vi "R=Table.vi"(6 "picture":refnum<vi>, 8 "Offset":T4, 9 "Matrix":T3 format="%.3f", 11 "Command":string="Save") -> (0 "error out":errorcluster, 2 "Joints":dbl[](array[numeric]), 3 "Pose Out":T3 format="%.3f")   [LabVIEW 2013]
uses:
  <vilib>/Analysis/Matrix/Datatypes/RealMatrix.ctl
  ROS/Code/SubVIs/BaxterSide.ctl
  Teach Locations.ctl
  ROS/Code/Console/Servers/ServerSubs/(nist) Arm Globals.vi
  Arm Globals.vi
  <vilib>/Analysis/baseanly.llb/Real Inverse Matrix.vi
  <vilib>/Analysis/Matrix/Numeric/Conversions/Array To Matrix - RA.vi
  <vilib>/Analysis/Matrix/Numeric/Multiply/Multiply - RM,RM.vi
  Move/Move XYA.vi
  <vilib>/Utility/config.llb/Write Key (String).vi
  <vilib>/Utility/config.llb/Read Key (String).vi
  <vilib>/Analysis/NI_AALBase.lvlib
  <vilib>/Analysis/Matrix/NI_Matrix.lvlib
  <vilib>/Utility/config.llb/NI_LVConfig.lvlib
panel:
  in  "Tab Control":T1(tab)=enum."Calibration Table"
  out "picture 2":picture
  out "Progress":T2
  out "IK Found":bool=TRUE
  in  "Table":T5={"Far Left"={"Absolute"=[250.0, 545.0, 0.0, 0.0], "Robot"=[672.1715994990807, 48.007748317552725, 100.0, 20.0]}, "Far Right"={"Absolute"=[250.0, 25.0, 0.0, 0.0], "Robot"=[665.1874122546096, -469.0278466112149, 100.0, 20.0]}, "Near Left"={"Absolute"=[25.0, 545.0, 0.0, 0.0], "Robot"=[441.4908301445158, 48.901036437406674, 100.0, 20.0]}, "Near Right"={"Absolute"=[25.0, 25.0, 0.0, 0.0], "Robot"=[437.9607504937842, -467.7872050538727, 100.0, 20.0]}}
  in  "Reference":dbl[](array[numeric])=[44.89013666745554, -43.242187450588595, -0.1098632811244629, 63.3471678963653, 0.1318359373493555, 69.71923820158416, -0.021972656224892577]
  # "Basic Commands are:\n   Convert   - convert offset to joints\n   Current   - current joint and offset\n   Register  - determine position\n   Save      - save calibration data\n   Load      - load calibration data\n   Reference - give reference joint position"
  # "Position gripper over center before starting"
  # "Insert the Absolute Positions here before \nrunning registration\n\nRun \"Save\" to load this table.\nMust manual set current values to default\nand save the vi."
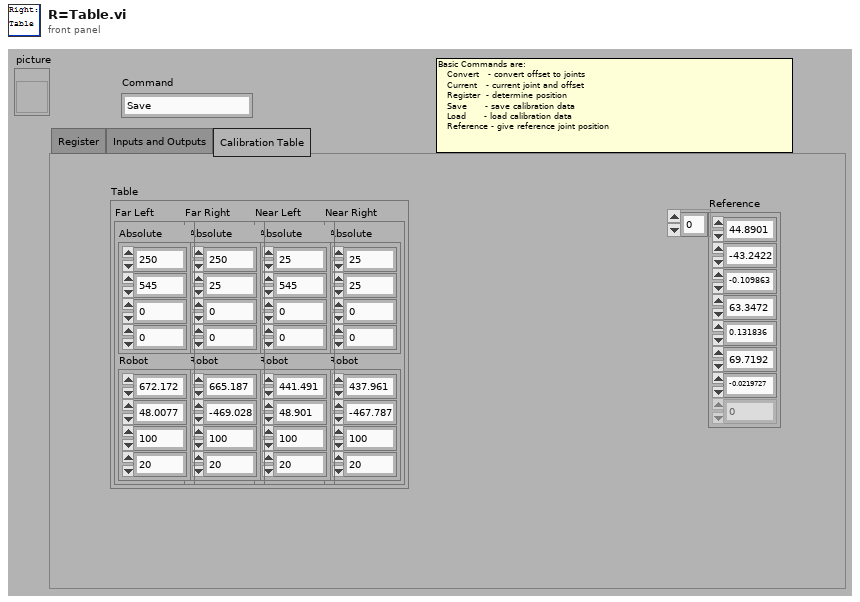
[diagram p1: front panel]
types:
  T1 = enum32{"Register", "Inputs and Outputs", "Calibration Table"}
  T2 = cluster{"1":bool, "1 2":bool, "1 3":bool, "1 4":bool}
  T3 = typedef "NI_Matrix.lvlib/RealMatrix.ctl" = dbl[][]
  T4 = cluster{"X":dbl, "Y":dbl, "Z":dbl, "Roll":dbl, "Pitch":dbl, "Yaw":dbl}
  T5 = cluster{"Far Left":cluster{"Absolute":dbl[], "Robot":dbl[]}, "Far Right":cluster{"Absolute":dbl[], "Robot":dbl[]}, "Near Left":cluster{"Absolute":dbl[], "Robot":dbl[]}, "Near Right":cluster{"Absolute":dbl[], "Robot":dbl[]}}
  T6 = typedef "BaxterSide.ctl" = enum16{"left", "right"}
  T7 = typedef "Teach Locations.ctl" = enum16{"Far_Right", "Near_Right", "Far_Left", "Near_Left", "Bottom", "Top", "Right", "Left"}
  T8 = typedef "NI_LVConfig.lvlib/Config Data RefNum.ctl" = refnum<k1>
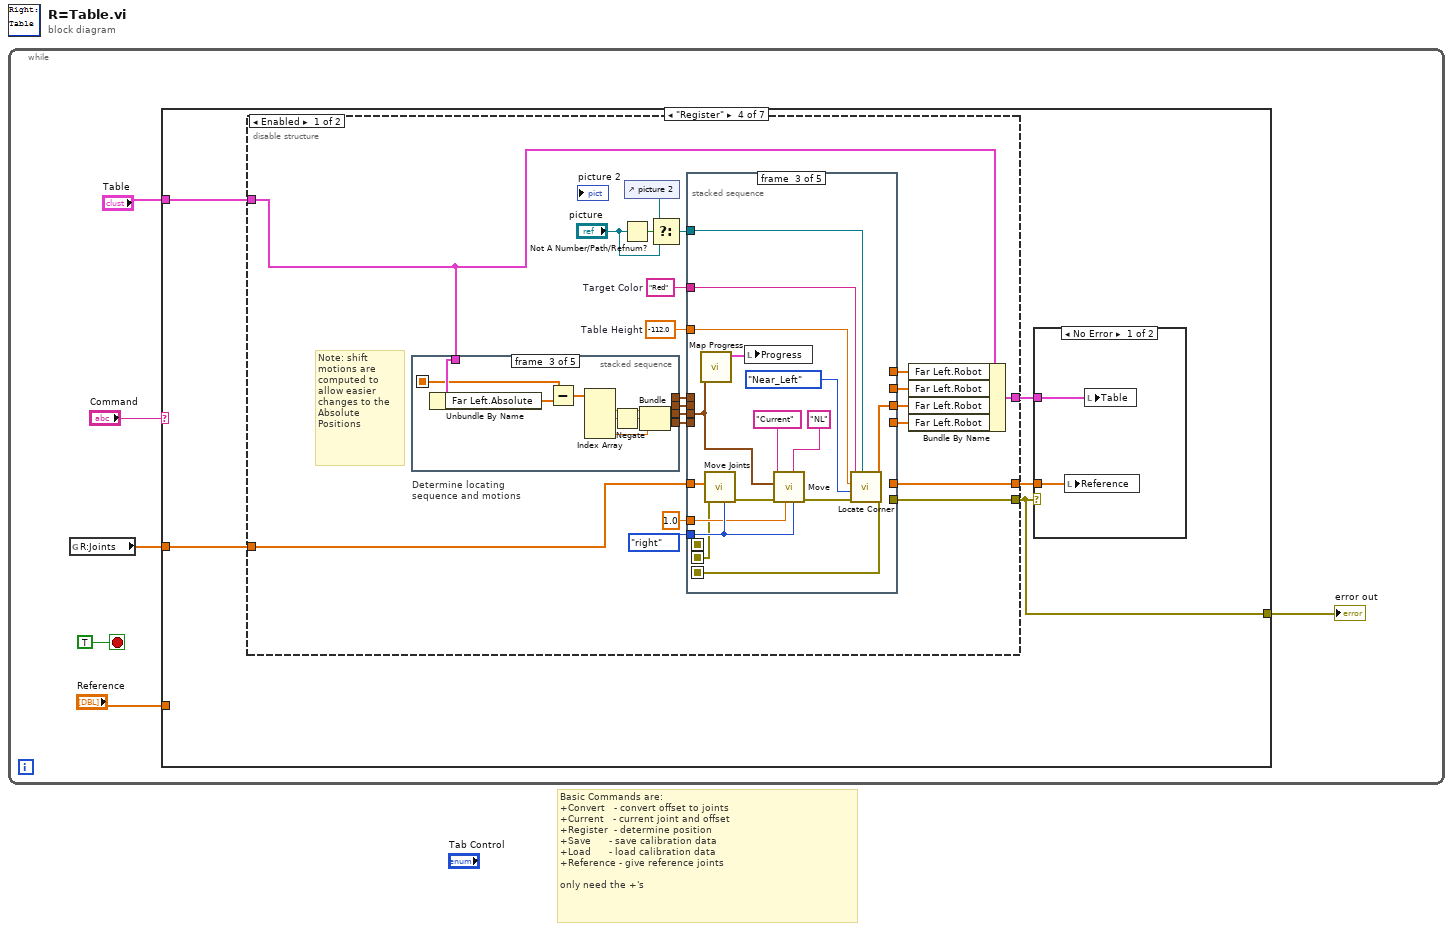
[diagram p0: block diagram]
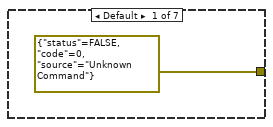
[diagram p2: hidden frame]
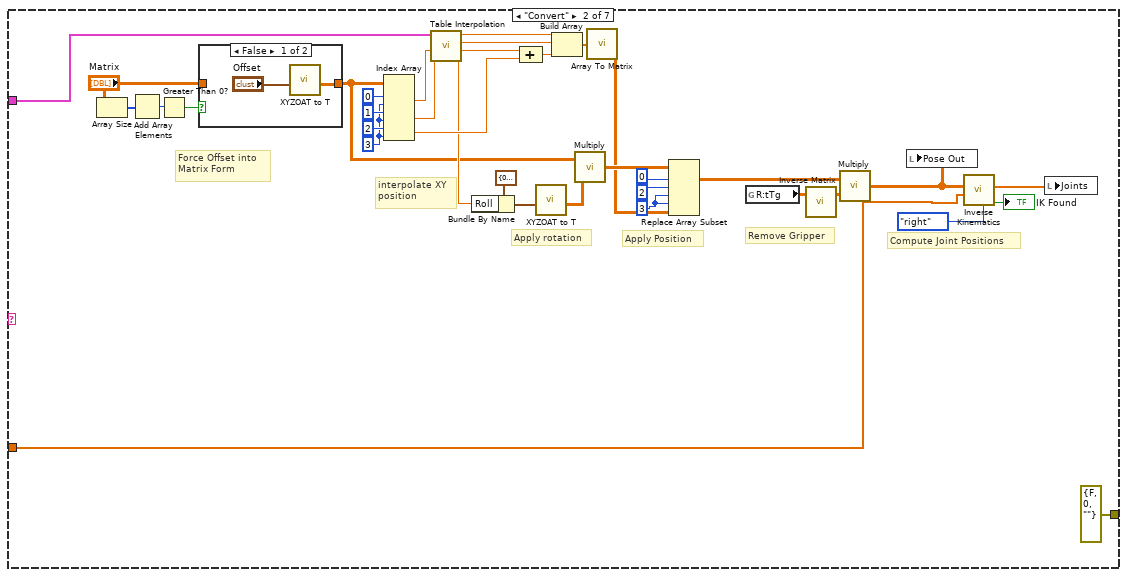
[diagram p3: hidden frame]
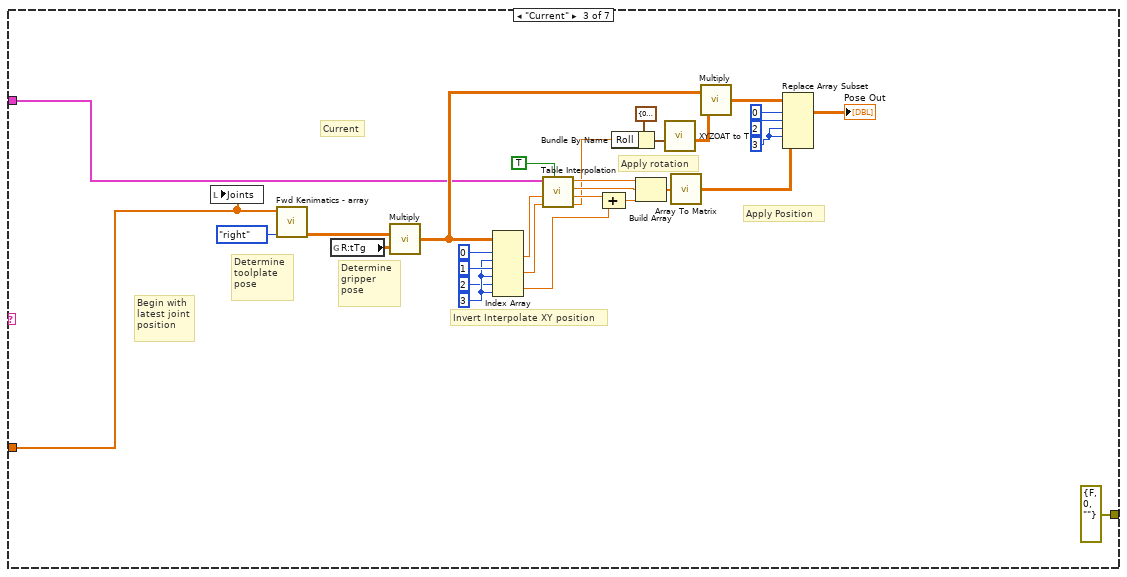
[diagram p5: hidden frame]
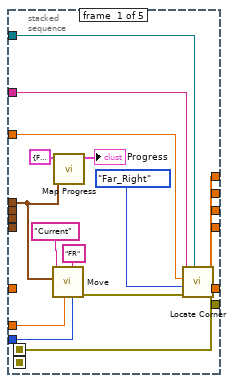
[diagram p6: hidden frame]
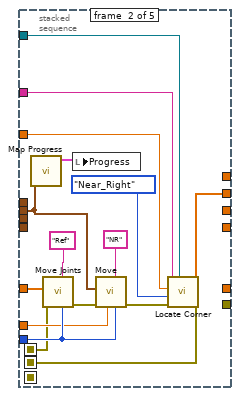
[diagram p7: hidden frame]
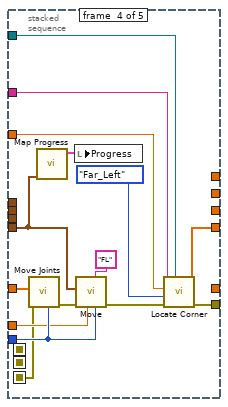
[diagram p8: hidden frame]
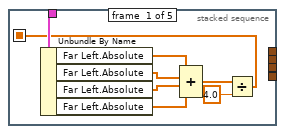
[diagram p10: hidden frame]
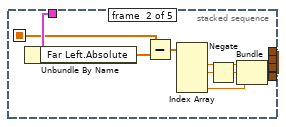
[diagram p11: hidden frame]
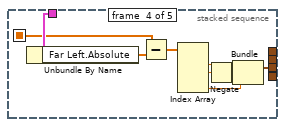
[diagram p12: hidden frame]
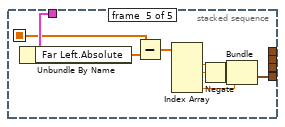
[diagram p13: hidden frame]
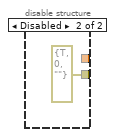
[diagram p14: hidden frame]
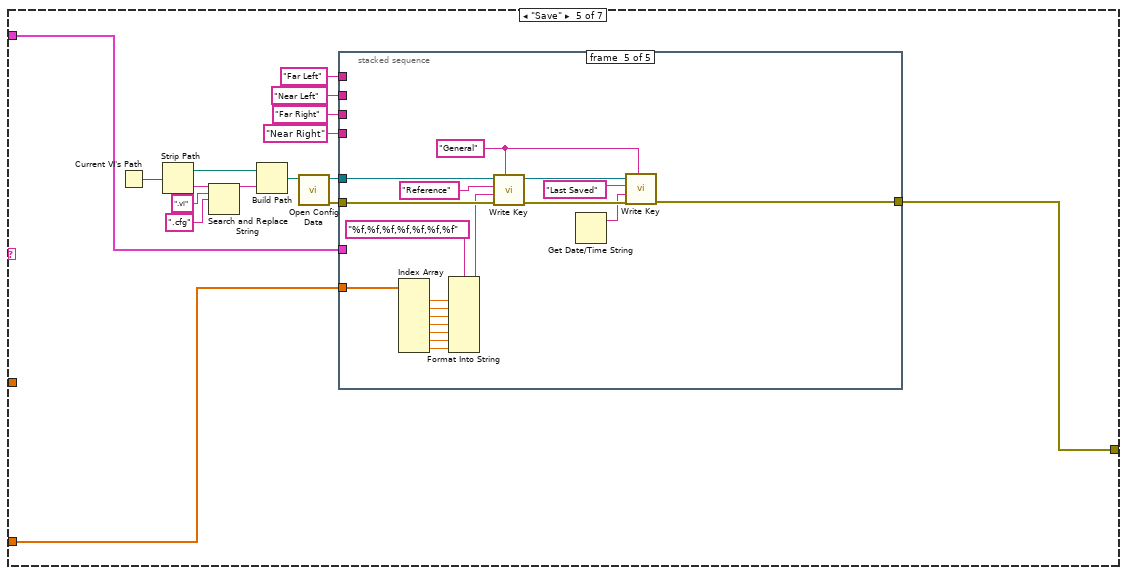
[diagram p16: hidden frame]
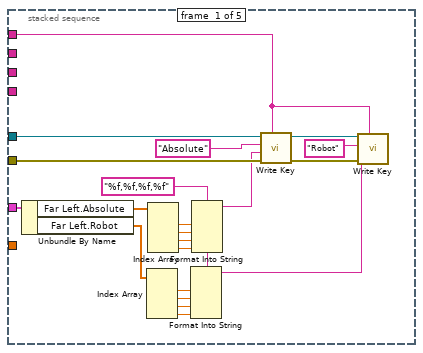
[diagram p17: hidden frame]
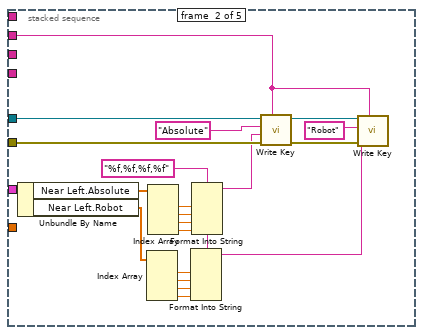
[diagram p18: hidden frame]
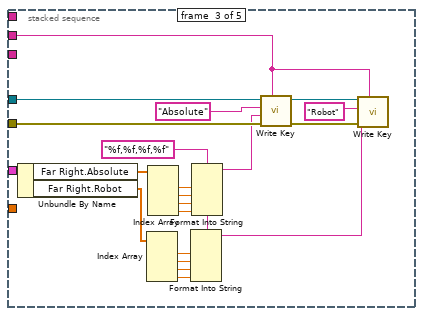
[diagram p19: hidden frame]
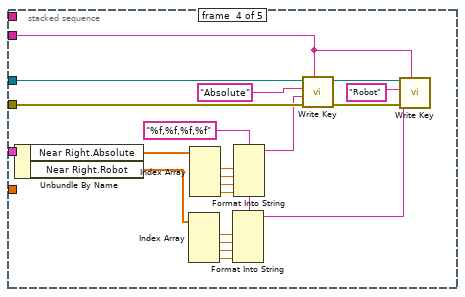
[diagram p20: hidden frame]
diagram:
  # "Basic Commands are:\n+Convert   - convert offset to joints\n+Current   - current joint and offset\n+Register  - determine position\n+Save      - save calibration data\n+Load      - load calibration data\n+Reference - give reference joints\n\nonly need the +'s"
  n1 = while {
    stop <- TRUE stop-if-true
    n2 = global read "(nist) Arm Globals.vi" "R:Joints"() -> (w4:dbl[])
    n3 = case shown="\"Register\"" "Command" {
      tunnel: "Reference" -> [_ _ _ _ w212 _ w453]
      tunnel: w4 -> [_ w10 w49 w79 _ _ _]
      tunnel: "Table" -> [_ w9 w48 w78 w214 w334 _]
      tunnel: [errorcluster {"status"=FALSE, "code"=0, "source"="Unknown Command"} ("error out") errorcluster {"status"=FALSE, "code"=0, "source"=""} ("error out") errorcluster {"status"=FALSE, "code"=0, "source"=""} ("error out") w77 w213 w331 errorcluster {"status"=FALSE, "code"=0, "source"=""} ("error out")] -> w2
      frame Default {
      }
      frame "Convert" {
        w17 = 3 ("index (row)")
        w40 = 3 ("index (col)")
        # "Apply Position"
        # "Compute Joint Positions"
        # "Remove Gripper"
        # "Apply rotation"
        # "interpolate XY \nposition"
        # "Force Offset into \nMatrix Form"
        n4 = Array Size(array="Matrix") -> (size(s)=w29:i32[])
        n5 = Add Array Elements(numeric array=w29) -> (sum=w30:i32)
        n6 = Greater Than 0?(x=w30) -> (x > 0?=w28:bool)
        n7 = case shown="False" w28 {
          tunnel: "Matrix" -> [_ w46]
          tunnel: [w44 w46] -> w23
          frame False {
            n8 = call "XYZOAT to T.vi"("XYZOAT"="Offset") -> ("T"=w44:T3)  [unwired: 10 in]
          }
          frame True {
          }
        }
        n9 = Index Array(array=w23, index (row) #1=0 ("index (row)"), index (col) #1=w40, index (row) #2=1 ("index (row)"), index (col) #2=w40, index (row) #3=2 ("index (row)"), index (col) #3=w40) -> (element #1=w25:dbl, element #2=w26:dbl, element #3=w37:dbl)
        n10 = call "Table Interpolation.vi"("Y"=w26, "X"=w25, "Location"=w9) -> ("a"=w35:dbl, "z"=w38:dbl, "y"=w15:dbl, "x"=w16:dbl)  [unwired: 5 in]
        n11 = Bundle By Name(cluster=T4 {"X"=0.0, "Y"=0.0, "Z"=0.0, "Roll"=0.0, "Pitch"=0.0, "Yaw"=0.0} ("XYZOAT"), "Roll"=w35) -> (w36:T4)
        n12 = Compound Arithmetic op=ADD(w38, w37) -> (w14:dbl)
        n13 = call "XYZOAT to T.vi"("XYZOAT"=w36) -> ("T"=w22:T3)  [unwired: 10 in]
        n14 = Build Array(w16, w15, w14) -> (w13:dbl[])
        n15 = call-poly <vilib>:"Multiply.vi"("Real Matrix B"=w22, "Real Matrix A"=w23) -> ("A * B"=w21:T3)
        n16 = call-poly <vilib>:"Array To Matrix.vi"("Real 1D Array"=w13) -> ("Real Matrix (Column Vector)"=w12:T3)
        n17 = Replace Array Subset(array=w21, new element=w12, index (dim 0)=0 ("index (row)"), index (dim 1)=2 ("index (row)"), index (dim 2)=w17, index (dim 3)=w17) -> (w20:T3)
        n18 = global read "Arm Globals.vi" "R:tTg"() -> (w33:T3)
        n19 = call-poly <vilib>:"Inverse Matrix.vi"("Input Matrix"=w33) -> ("Inverse Matrix"=w34:T3)  [unwired: 1 in, 1 out]
        n20 = call-poly <vilib>:"Multiply.vi"("Real Matrix B"=w34, "Real Matrix A"=w20) -> ("A * B"=w24:T3)
        n21 = local write "Pose Out"(w24) -> ()
        n22 = call "Inverse Kinematics.vi"("Side"=BaxterSide."right", "Start"=w10, "Goal-matrix"=w24) -> ("Found"=→"IK Found":bool, "J"=w31:dbl[])  [unwired: 5 in, 2 out]
        n23 = local write "Joints"(w31) -> ()
      }
      frame "Current" {
        w54 = 3 ("index (row)")
        w68 = 3 ("index (col)")
        # "Apply Position"
        # "Apply rotation"
        # "Invert Interpolate XY position"
        # "Determine \ngripper\npose"
        # "Determine \ntoolplate\npose"
        # "Begin with\nlatest joint\nposition"
        # "Current"
        n24 = local write "Joints"(w49) -> ()
        n25 = call "Fwd Kenimatics - array.vi"("Side"=BaxterSide."right", "Joints"=w49) -> ("Matrix"=w73:T3)  [unwired: 8 in, 1 out]
        n26 = global read "Arm Globals.vi" "R:tTg"() -> (w74:T3)
        n27 = call-poly <vilib>:"Multiply.vi"("Real Matrix B"=w74, "Real Matrix A"=w73) -> ("A * B"=w58:T3)
        n28 = Index Array(array=w58, index (row) #1=0 ("index (row)"), index (col) #1=w68, index (row) #2=1 ("index (row)"), index (col) #2=w68, index (row) #3=2 ("index (col)"), index (col) #3=w68) -> (element #1=w70:dbl, element #2=w69:dbl, element #3=w65:dbl)
        n29 = call "Table Interpolation.vi"("Invert"=TRUE, "Y"=w69, "X"=w70, "Location"=w48) -> ("a"=w50:dbl, "z"=w66:dbl, "y"=w60:dbl, "x"=w61:dbl)  [unwired: 4 in]
        n30 = Compound Arithmetic op=ADD(w66, w65) -> (w59:dbl)
        n31 = Bundle By Name(cluster=T4 {"X"=0.0, "Y"=0.0, "Z"=0.0, "Roll"=0.0, "Pitch"=0.0, "Yaw"=0.0} ("XYZOAT"), "Roll"=w50) -> (w63:T4)
        n32 = Build Array(w61, w60, w59) -> (w62:dbl[])
        n33 = call "XYZOAT to T.vi"("XYZOAT"=w63) -> ("T"=w57:T3)  [unwired: 10 in]
        n34 = call-poly <vilib>:"Array To Matrix.vi"("Real 1D Array"=w62) -> ("Real Matrix (Column Vector)"=w51:T3)
        n35 = call-poly <vilib>:"Multiply.vi"("Real Matrix B"=w57, "Real Matrix A"=w58) -> ("A * B"=w53:T3)
        n36 = Replace Array Subset(array=w53, new element=w51, index (dim 0)=0 ("index (row)"), index (dim 1)=2 ("index (row)"), index (dim 2)=w54, index (dim 3)=w54) -> (→"Pose Out":T3)
      }
      frame "Register" {
        n37 = disable-structure shown="Enabled" {
          disable-tunnel: [w86 errorcluster {"status"=TRUE, "code"=0, "source"=""} ("error out")] -> w77
          disable-tunnel: [w85 _] -> w81
          disable-tunnel: [w84 _] -> w80
          disable-tunnel: w79 -> [w83 _]
          disable-tunnel: w78 -> [w82 _]
          frame Enabled {
            w101 = "Red"  # Target Color
            w96 = -112.0  # Table Height
            # "Note: shift motions are computed to allow easier\nchanges to the Absolute Positions"
            n38 = stacked-sequence "Determine locating sequence and motions" {
              seq-local: [w165 _ _ _ _] -> [_ w179 w188 w197 w206]
              tunnel: w82 -> [w172 w181 w190 w199 w208]
              tunnel: [_ _ w183 _ _] -> w100
              tunnel: [_ _ _ w192 _] -> w99
              tunnel: [_ _ _ _ w201] -> w98
              tunnel: [_ w174 _ _ _] -> w97
              frame #0 {
                n39 = Unbundle By Name(w172) -> ("Far Left.Absolute"=w171:dbl[], "Far Left.Absolute"=w170:dbl[], "Far Left.Absolute"=w169:dbl[], "Far Left.Absolute"=w168:dbl[])
                n40 = Compound Arithmetic op=ADD(w171, w170, w169, w168) -> (w167:dbl[])
                n41 = Divide(x=w167, y=4.0) -> (x/y=w165:dbl[])
              }
              frame #1 {
                n42 = Unbundle By Name(w181) -> ("Far Left.Absolute"=w180:dbl[])
                n43 = Subtract(x=w179, y=w180) -> (x-y=w178:dbl[])
                n44 = Index Array(array=w178) -> (element #1=w176:dbl, element #2=w177:dbl, element #4=w175:dbl)  [unwired: 4 in, 1 out]
                n45 = Negate(x=w177) -> (-x=w173:dbl)
                n46 = Bundle(w176, w173, w175) -> (w174:cluster{dbl, dbl, dbl})  [unwired: 1 in]
              }
              frame #2 {
                n47 = Unbundle By Name(w190) -> ("Far Left.Absolute"=w189:dbl[])
                n48 = Subtract(x=w188, y=w189) -> (x-y=w187:dbl[])
                n49 = Index Array(array=w187) -> (element #1=w185:dbl, element #2=w186:dbl, element #4=w184:dbl)  [unwired: 4 in, 1 out]
                n50 = Negate(x=w186) -> (-x=w182:dbl)
                n51 = Bundle(w185, w182, w184) -> (w183:cluster{dbl, dbl, dbl})  [unwired: 1 in]
              }
              frame #3 {
                n52 = Unbundle By Name(w199) -> ("Far Left.Absolute"=w198:dbl[])
                n53 = Subtract(x=w197, y=w198) -> (x-y=w196:dbl[])
                n54 = Index Array(array=w196) -> (element #1=w194:dbl, element #2=w195:dbl, element #4=w193:dbl)  [unwired: 4 in, 1 out]
                n55 = Negate(x=w195) -> (-x=w191:dbl)
                n56 = Bundle(w194, w191, w193) -> (w192:cluster{dbl, dbl, dbl})  [unwired: 1 in]
              }
              frame #4 {
                n57 = Unbundle By Name(w208) -> ("Far Left.Absolute"=w207:dbl[])
                n58 = Subtract(x=w206, y=w207) -> (x-y=w205:dbl[])
                n59 = Index Array(array=w205) -> (element #1=w203:dbl, element #2=w204:dbl, element #4=w202:dbl)  [unwired: 4 in, 1 out]
                n60 = Negate(x=w204) -> (-x=w200:dbl)
                n61 = Bundle(w203, w200, w202) -> (w201:cluster{dbl, dbl, dbl})  [unwired: 1 in]
              }
            }
            n62 = Not A Number/Path/Refnum?(number/path/refnum="picture") -> (NaN/Path/Refnum?=w95:bool)
            n63 = control-ref of="picture 2"() -> (w93:refnum<vi>)
            n64 = Select(t=w93, s=w95, f="picture") -> (s? t:f=w102:refnum<vi>)
            n65 = stacked-sequence {
              seq-local: [w108 _ _ _ _] -> [_ w123 _ _ _]
              seq-local: [_ w122 _ _ _] -> [_ _ w140 _ _]
              seq-local: [_ _ w139 _ _] -> [_ _ _ w153 _]
              tunnel: w101 -> [w114 w128 w146 w160 _]
              tunnel: w100 -> [_ w118 _ _ _]
              tunnel: [_ w127 _ _ _] -> w92
              tunnel: w102 -> [w113 w126 w145 w159 _]
              tunnel: w83 -> [_ w121 w137 w152 w164]
              tunnel: BaxterSide."right" ("Side") -> [w112 w125 w144 w158 _]
              tunnel: [_ _ w143 _ _] -> w91
              tunnel: w99 -> [_ _ w135 _ _]
              tunnel: w97 -> [w106 _ _ _ _]
              tunnel: [w110 _ _ _ _] -> w90
              tunnel: [_ _ _ w156 _] -> w89
              tunnel: w98 -> [_ _ _ w151 _]
              tunnel: [_ _ _ w155 _] -> w86
              tunnel: 1.0 ("wait time") -> [w109 w124 w141 w154 _]
              tunnel: w96 -> [w103 w117 w133 w149 _]
              tunnel: [_ _ _ _ w164] -> w84
              frame #0 {
                n66 = call-poly "Move.vi"("Side"=w112, "Label"="FR", "Wait Time"=w109, "XYA"=w106, "Location"="Current") -> ("error out"=w115:errorcluster)  [unwired: 6 in]
                n67 = call "Map Progress.vi"("Shift"=w106, "Cluster"=T2 {"1"=FALSE, "1 2"=FALSE, "1 3"=FALSE, "1 4"=FALSE}) -> ("Cluster 2"=→"Progress":T2)  [unwired: 9 in]
                n68 = call "Locate Corner.vi"("picture"=w113, "error in"=w115, "Corner Type"=Teach_Locations."Far_Right" ("Feature"), "Height"=w103, "color"=w114) -> ("error out"=w108:errorcluster, "Robot Point"=w110:dbl[])  [unwired: 4 in, 1 out]
              }
              frame #1 {
                n69 = call "Map Progress.vi"("Shift"=w118) -> ("Cluster 2"=w119:T2)  [unwired: 10 in]
                n70 = call "Move Joints.vi"("Side"=w125, "Label"="Ref", "error in"=w123, "Goal"=w121) -> ("error out"=w132:errorcluster)  [unwired: 6 in, 1 out]
                n71 = local write "Progress"(w119) -> ()
                n72 = call-poly "Move.vi"("Side"=w125, "Label"="NR", "Wait Time"=w124, "error in"=w132, "XYA"=w118) -> ("error out"=w130:errorcluster)  [unwired: 6 in]
                n73 = call "Locate Corner.vi"("picture"=w126, "error in"=w130, "Corner Type"=Teach_Locations."Near_Right", "Height"=w117, "color"=w128) -> ("error out"=w122:errorcluster, "Robot Point"=w127:dbl[])  [unwired: 4 in, 1 out]
              }
              frame #2 {
                n74 = call "Map Progress.vi"("Shift"=w135) -> ("Cluster 2"=w134:T2)  [unwired: 10 in]
                n75 = call "Move Joints.vi"("Side"=w144, "error in"=w140, "Goal"=w137) -> ("error out"=w148:errorcluster)  [unwired: 7 in, 1 out]
                n76 = local write "Progress"(w134) -> ()
                n77 = call-poly "Move.vi"("Side"=w144, "Label"="NL", "Wait Time"=w141, "error in"=w148, "XYA"=w135, "Location"="Current") -> ("error out"=w147:errorcluster)  [unwired: 5 in]
                n78 = call "Locate Corner.vi"("picture"=w145, "error in"=w147, "Corner Type"=Teach_Locations."Near_Left", "Height"=w133, "color"=w146) -> ("error out"=w139:errorcluster, "Robot Point"=w143:dbl[])  [unwired: 4 in, 1 out]
              }
              frame #3 {
                n79 = call "Move Joints.vi"("Side"=w158, "error in"=w153, "Goal"=w152) -> ("error out"=w163:errorcluster)  [unwired: 7 in, 1 out]
                n80 = call "Map Progress.vi"("Shift"=w151) -> ("Cluster 2"=w150:T2)  [unwired: 10 in]
                n81 = local write "Progress"(w150) -> ()
                n82 = call-poly "Move.vi"("Side"=w158, "Label"="FL", "Wait Time"=w154, "error in"=w163, "XYA"=w151) -> ("error out"=w161:errorcluster)  [unwired: 6 in]
                n83 = call "Locate Corner.vi"("picture"=w159, "error in"=w161, "Corner Type"=Teach_Locations."Far_Left", "Height"=w149, "color"=w160) -> ("error out"=w155:errorcluster, "Robot Point"=w156:dbl[])  [unwired: 4 in, 1 out]
              }
              frame #4 {
              }
            }
            n84 = Bundle By Name(cluster=w82, "Far Left.Robot"=w90, "Far Left.Robot"=w92, "Far Left.Robot"=w91, "Far Left.Robot"=w89) -> (w85:T5)
          }
          frame Disabled {
          }
        }
        n85 = case shown="No Error" w77 {
          tunnel: w81 -> [w211 _]
          tunnel: w80 -> [w210 _]
          frame No Error {
            n86 = local write "Reference"(w210) -> ()
            n87 = local write "Table"(w211) -> ()
          }
          frame Error {
          }
        }
      }
      frame "Save" {
        n88 = Current VI's Path() -> (path=w225:path)
        n89 = Strip Path(path=w225) -> (stripped path=w220:path, name=w224:string)
        n90 = Search and Replace String(input string=w224, search string=".vi", replace string=".cfg" ("replace string (\"\")")) -> (result string=w221:string)  [unwired: 5 in, 3 out]
        n91 = Build Path(base path=w220, name or relative path=w221) -> (appended path=w219:path)
        n92 = call <vilib>:"Open Config Data.vi"("configuration file path"=w219) -> ("error out"=w226:errorcluster, "refnum"=w227:T8)  [unwired: 8 in, 1 out]
        n93 = stacked-sequence {
          tunnel: w227 -> [w248 w269 w290 w311 w330]
          tunnel: w226 -> [w247 w268 w289 w310 w329]
          tunnel: w214 -> [w245 w266 w287 w308 _]
          tunnel: "Far Left" ("section") -> [w228 _ _ _ _]
          tunnel: "Near Left" ("section") -> [_ w249 _ _ _]
          tunnel: "Far Right" ("section") -> [_ _ w270 _ _]
          tunnel: "Near Right" ("section") -> [_ _ _ w291 _]
          tunnel: w212 -> [_ _ _ _ w326]
          tunnel: [_ _ _ _ w312] -> w213
          frame #0 {
            w231 = "%f,%f,%f,%f" ("format string")
            n94 = Unbundle By Name(w245) -> ("Far Left.Absolute"=w244:dbl[], "Far Left.Robot"=w230:dbl[])
            n95 = Index Array(array=w230) -> (element #1=w235:dbl, element #2=w234:dbl, element #3=w233:dbl, element #4=w232:dbl)  [unwired: 4 in]
            n96 = Index Array(array=w244) -> (element #1=w243:dbl, element #2=w242:dbl, element #3=w241:dbl, element #4=w240:dbl)  [unwired: 4 in]
            n97 = Format Into String(format string=w231, w235, w234, w233, w232) -> (resulting string=w229:string)  [unwired: 2 in, 1 out]
            n98 = Format Into String(format string=w231, w243, w242, w241, w240) -> (resulting string=w239:string)  [unwired: 2 in, 1 out]
            n99 = call-poly <vilib>:"Write Key.vi"("section"=w228, "error in (no error)"=w247, "value"=w239, "key"="Absolute", "refnum"=w248) -> ("error out"=w237:errorcluster, "refnum out"=w238:T8)  [unwired: 4 in, 1 out]
            n100 = call-poly <vilib>:"Write Key.vi"("section"=w228, "error in (no error)"=w237, "value"=w229, "key"="Robot", "refnum"=w238) -> ()  [unwired: 4 in, 3 out]
          }
          frame #1 {
            w252 = "%f,%f,%f,%f" ("format string")
            n101 = Unbundle By Name(w266) -> ("Near Left.Absolute"=w265:dbl[], "Near Left.Robot"=w251:dbl[])
            n102 = Index Array(array=w251) -> (element #1=w256:dbl, element #2=w255:dbl, element #3=w254:dbl, element #4=w253:dbl)  [unwired: 4 in]
            n103 = Index Array(array=w265) -> (element #1=w264:dbl, element #2=w263:dbl, element #3=w262:dbl, element #4=w261:dbl)  [unwired: 4 in]
            n104 = Format Into String(format string=w252, w256, w255, w254, w253) -> (resulting string=w250:string)  [unwired: 2 in, 1 out]
            n105 = Format Into String(format string=w252, w264, w263, w262, w261) -> (resulting string=w260:string)  [unwired: 2 in, 1 out]
            n106 = call-poly <vilib>:"Write Key.vi"("section"=w249, "error in (no error)"=w268, "value"=w260, "key"="Absolute", "refnum"=w269) -> ("error out"=w258:errorcluster, "refnum out"=w259:T8)  [unwired: 4 in, 1 out]
            n107 = call-poly <vilib>:"Write Key.vi"("section"=w249, "error in (no error)"=w258, "value"=w250, "key"="Robot", "refnum"=w259) -> ()  [unwired: 4 in, 3 out]
          }
          frame #2 {
            w273 = "%f,%f,%f,%f" ("format string")
            n108 = Unbundle By Name(w287) -> ("Far Right.Absolute"=w286:dbl[], "Far Right.Robot"=w272:dbl[])
            n109 = Index Array(array=w272) -> (element #1=w277:dbl, element #2=w276:dbl, element #3=w275:dbl, element #4=w274:dbl)  [unwired: 4 in]
            n110 = Index Array(array=w286) -> (element #1=w285:dbl, element #2=w284:dbl, element #3=w283:dbl, element #4=w282:dbl)  [unwired: 4 in]
            n111 = Format Into String(format string=w273, w277, w276, w275, w274) -> (resulting string=w271:string)  [unwired: 2 in, 1 out]
            n112 = Format Into String(format string=w273, w285, w284, w283, w282) -> (resulting string=w281:string)  [unwired: 2 in, 1 out]
            n113 = call-poly <vilib>:"Write Key.vi"("section"=w270, "error in (no error)"=w289, "value"=w281, "key"="Absolute", "refnum"=w290) -> ("error out"=w279:errorcluster, "refnum out"=w280:T8)  [unwired: 4 in, 1 out]
            n114 = call-poly <vilib>:"Write Key.vi"("section"=w270, "error in (no error)"=w279, "value"=w271, "key"="Robot", "refnum"=w280) -> ()  [unwired: 4 in, 3 out]
          }
          frame #3 {
            w294 = "%f,%f,%f,%f" ("format string")
            n115 = Unbundle By Name(w308) -> ("Near Right.Absolute"=w307:dbl[], "Near Right.Robot"=w293:dbl[])
            n116 = Index Array(array=w293) -> (element #1=w298:dbl, element #2=w297:dbl, element #3=w296:dbl, element #4=w295:dbl)  [unwired: 4 in]
            n117 = Index Array(array=w307) -> (element #1=w306:dbl, element #2=w305:dbl, element #3=w304:dbl, element #4=w303:dbl)  [unwired: 4 in]
            n118 = Format Into String(format string=w294, w298, w297, w296, w295) -> (resulting string=w292:string)  [unwired: 2 in, 1 out]
            n119 = Format Into String(format string=w294, w306, w305, w304, w303) -> (resulting string=w302:string)  [unwired: 2 in, 1 out]
            n120 = call-poly <vilib>:"Write Key.vi"("section"=w291, "error in (no error)"=w310, "value"=w302, "key"="Absolute", "refnum"=w311) -> ("error out"=w300:errorcluster, "refnum out"=w301:T8)  [unwired: 4 in, 1 out]
            n121 = call-poly <vilib>:"Write Key.vi"("section"=w291, "error in (no error)"=w300, "value"=w292, "key"="Robot", "refnum"=w301) -> ()  [unwired: 4 in, 3 out]
          }
          frame #4 {
            w315 = "General" ("section")
            n122 = Index Array(array=w326) -> (element #1=w325:dbl, element #2=w324:dbl, element #3=w323:dbl, element #4=w322:dbl, element #5=w321:dbl, element #6=w320:dbl, element #7=w319:dbl)  [unwired: 7 in]
            n123 = Format Into String(format string="%f,%f,%f,%f,%f,%f,%f", w325, w324, w323, w322, w321, w320, w319) -> (resulting string=w318:string)  [unwired: 2 in, 1 out]
            n124 = call-poly <vilib>:"Write Key.vi"("section"=w315, "error in (no error)"=w329, "value"=w318, "key"="Reference", "refnum"=w330) -> ("error out"=w316:errorcluster, "refnum out"=w317:T8)  [unwired: 4 in, 1 out]
            n125 = Get Date/Time String() -> (date string=w314:string)  [unwired: 3 in, 1 out]
            n126 = call-poly <vilib>:"Write Key.vi"("section"=w315, "error in (no error)"=w316, "value"=w314, "key"="Last Saved", "refnum"=w317) -> ("error out"=w312:errorcluster)  [unwired: 4 in, 2 out]
          }
        }
      }
      frame "Load" {
        n127 = Current VI's Path() -> (path=w353:path)
        n128 = Strip Path(path=w353) -> (stripped path=w348:path, name=w352:string)
        n129 = Search and Replace String(input string=w352, search string=".vi", replace string=".cfg" ("replace string (\"\")")) -> (result string=w349:string)  [unwired: 5 in, 3 out]
        n130 = Build Path(base path=w348, name or relative path=w349) -> (appended path=w347:path)
        n131 = call <vilib>:"Open Config Data.vi"("configuration file path"=w347) -> ("error out"=w354:errorcluster, "refnum"=w355:T8)  [unwired: 8 in, 1 out]
        n132 = stacked-sequence {
          tunnel: w355 -> [w375 w395 w415 w435 w451]
          tunnel: w354 -> [w374 w394 w414 w434 w450]
          tunnel: [_ _ _ _ w438] -> w332
          tunnel: [_ _ _ _ w436] -> w331
          tunnel: "Far Left" ("section") -> [w358 _ _ _ _]
          tunnel: [w357 _ _ _ _] -> w345
          tunnel: [w356 _ _ _ _] -> w344
          tunnel: "Near Left" ("section") -> [_ w378 _ _ _]
          tunnel: [_ w377 _ _ _] -> w342
          tunnel: [_ w376 _ _ _] -> w341
          tunnel: "Far Right" ("section") -> [_ _ w398 _ _]
          tunnel: [_ _ w397 _ _] -> w339
          tunnel: [_ _ w396 _ _] -> w338
          tunnel: "Near Right" ("section") -> [_ _ _ w418 _]
          tunnel: [_ _ _ w417 _] -> w336
          tunnel: [_ _ _ w416 _] -> w335
          frame #0 {
            w363 = "%f,%f,%f,%f" ("format string")
            n133 = call-poly <vilib>:"Read Key.vi"("section"=w358, "error in (no error)"=w374, "key"="Absolute", "refnum"=w375) -> ("error out"=w362:errorcluster, "value"=w372:string, "refnum out"=w361:T8)  [unwired: 4 in, 1 out]
            n134 = call-poly <vilib>:"Read Key.vi"("section"=w358, "error in (no error)"=w362, "key"="Robot", "refnum"=w361) -> ("value"=w359:string)  [unwired: 4 in, 3 out]
            n135 = Scan From String(format string=w363, input string=w372) -> (output 1=w371:dbl, output 2=w370:dbl, output 3=w369:dbl, output 4=w368:dbl)  [unwired: 6 in, 3 out]
            n136 = Scan From String(format string=w363, input string=w359) -> (output 1=w367:dbl, output 2=w366:dbl, output 3=w365:dbl, output 4=w364:dbl)  [unwired: 6 in, 3 out]
            n137 = Build Array(w371, w370, w369, w368) -> (w357:dbl[])
            n138 = Build Array(w367, w366, w365, w364) -> (w356:dbl[])
          }
          frame #1 {
            w383 = "%f,%f,%f,%f" ("format string")
            n139 = call-poly <vilib>:"Read Key.vi"("section"=w378, "error in (no error)"=w394, "key"="Absolute", "refnum"=w395) -> ("error out"=w382:errorcluster, "value"=w392:string, "refnum out"=w381:T8)  [unwired: 4 in, 1 out]
            n140 = call-poly <vilib>:"Read Key.vi"("section"=w378, "error in (no error)"=w382, "key"="Robot", "refnum"=w381) -> ("value"=w379:string)  [unwired: 4 in, 3 out]
            n141 = Scan From String(format string=w383, input string=w392) -> (output 1=w391:dbl, output 2=w390:dbl, output 3=w389:dbl, output 4=w388:dbl)  [unwired: 6 in, 3 out]
            n142 = Scan From String(format string=w383, input string=w379) -> (output 1=w387:dbl, output 2=w386:dbl, output 3=w385:dbl, output 4=w384:dbl)  [unwired: 6 in, 3 out]
            n143 = Build Array(w391, w390, w389, w388) -> (w377:dbl[])
            n144 = Build Array(w387, w386, w385, w384) -> (w376:dbl[])
          }
          frame #2 {
            w403 = "%f,%f,%f,%f" ("format string")
            n145 = call-poly <vilib>:"Read Key.vi"("section"=w398, "error in (no error)"=w414, "key"="Absolute", "refnum"=w415) -> ("error out"=w402:errorcluster, "value"=w412:string, "refnum out"=w401:T8)  [unwired: 4 in, 1 out]
            n146 = call-poly <vilib>:"Read Key.vi"("section"=w398, "error in (no error)"=w402, "key"="Robot", "refnum"=w401) -> ("value"=w399:string)  [unwired: 4 in, 3 out]
            n147 = Scan From String(format string=w403, input string=w412) -> (output 1=w411:dbl, output 2=w410:dbl, output 3=w409:dbl, output 4=w408:dbl)  [unwired: 6 in, 3 out]
            n148 = Scan From String(format string=w403, input string=w399) -> (output 1=w407:dbl, output 2=w406:dbl, output 3=w405:dbl, output 4=w404:dbl)  [unwired: 6 in, 3 out]
            n149 = Build Array(w411, w410, w409, w408) -> (w397:dbl[])
            n150 = Build Array(w407, w406, w405, w404) -> (w396:dbl[])
          }
          frame #3 {
            w423 = "%f,%f,%f,%f" ("format string")
            n151 = call-poly <vilib>:"Read Key.vi"("section"=w418, "error in (no error)"=w434, "key"="Absolute", "refnum"=w435) -> ("error out"=w422:errorcluster, "value"=w432:string, "refnum out"=w421:T8)  [unwired: 4 in, 1 out]
            n152 = call-poly <vilib>:"Read Key.vi"("section"=w418, "error in (no error)"=w422, "key"="Robot", "refnum"=w421) -> ("value"=w419:string)  [unwired: 4 in, 3 out]
            n153 = Scan From String(format string=w423, input string=w432) -> (output 1=w431:dbl, output 2=w430:dbl, output 3=w429:dbl, output 4=w428:dbl)  [unwired: 6 in, 3 out]
            n154 = Scan From String(format string=w423, input string=w419) -> (output 1=w427:dbl, output 2=w426:dbl, output 3=w425:dbl, output 4=w424:dbl)  [unwired: 6 in, 3 out]
            n155 = Build Array(w431, w430, w429, w428) -> (w417:dbl[])
            n156 = Build Array(w427, w426, w425, w424) -> (w416:dbl[])
          }
          frame #4 {
            w437 = 360.0 ("default value 1")
            n157 = call-poly <vilib>:"Read Key.vi"("section"="General", "error in (no error)"=w450, "key"="Reference", "refnum"=w451) -> ("error out"=w436:errorcluster, "value"=w448:string)  [unwired: 4 in, 2 out]
            n158 = Scan From String(format string="%f,%f,%f,%f,%f,%f,%f", input string=w448, default 1=w437, default 2=w437, default 3=w437, default 4=w437, default 5=w437, default 6=w437, default 7=w437) -> (output 1=w447:dbl, output 2=w446:dbl, output 3=w445:dbl, output 4=w444:dbl, output 5=w441:dbl, output 6=w440:dbl, output 7=w439:dbl)  [unwired: 2 in, 3 out]
            n159 = Build Array(w447, w446, w445, w444, w441, w440, w439) -> (w438:dbl[])
          }
        }
        n160 = Bundle By Name(cluster=w334, "Far Left.Absolute"=w345, "Far Left.Robot"=w344, "Far Left.Absolute"=w342, "Near Left.Robot"=w341, "Far Right.Absolute"=w339, "Far Right.Robot"=w338, "Near Right.Absolute"=w336, "Near Right.Robot"=w335) -> (w333:T5)
        n161 = local write "Reference"(w332) -> ()
        n162 = local write "Table"(w333) -> ()
      }
      frame "Reference" {
        "Joints" <- w453
      }
    }
    "error out" <- w2
  }
